vi "GPS.vi"(0 "String":string) -> (1 "Hora":string, 2 "Ubicación":string, 3 "Velocidad":string, 4 "Fecha":string)   [LabVIEW 2020]
doc: "Este programa desglosa las tramas rmc"
panel:
  out "A or V":string
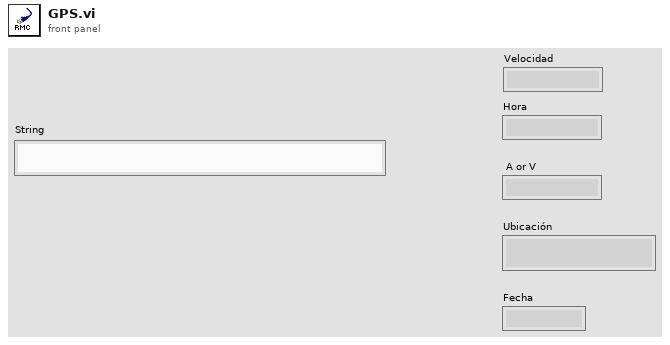
[diagram p1: front panel]
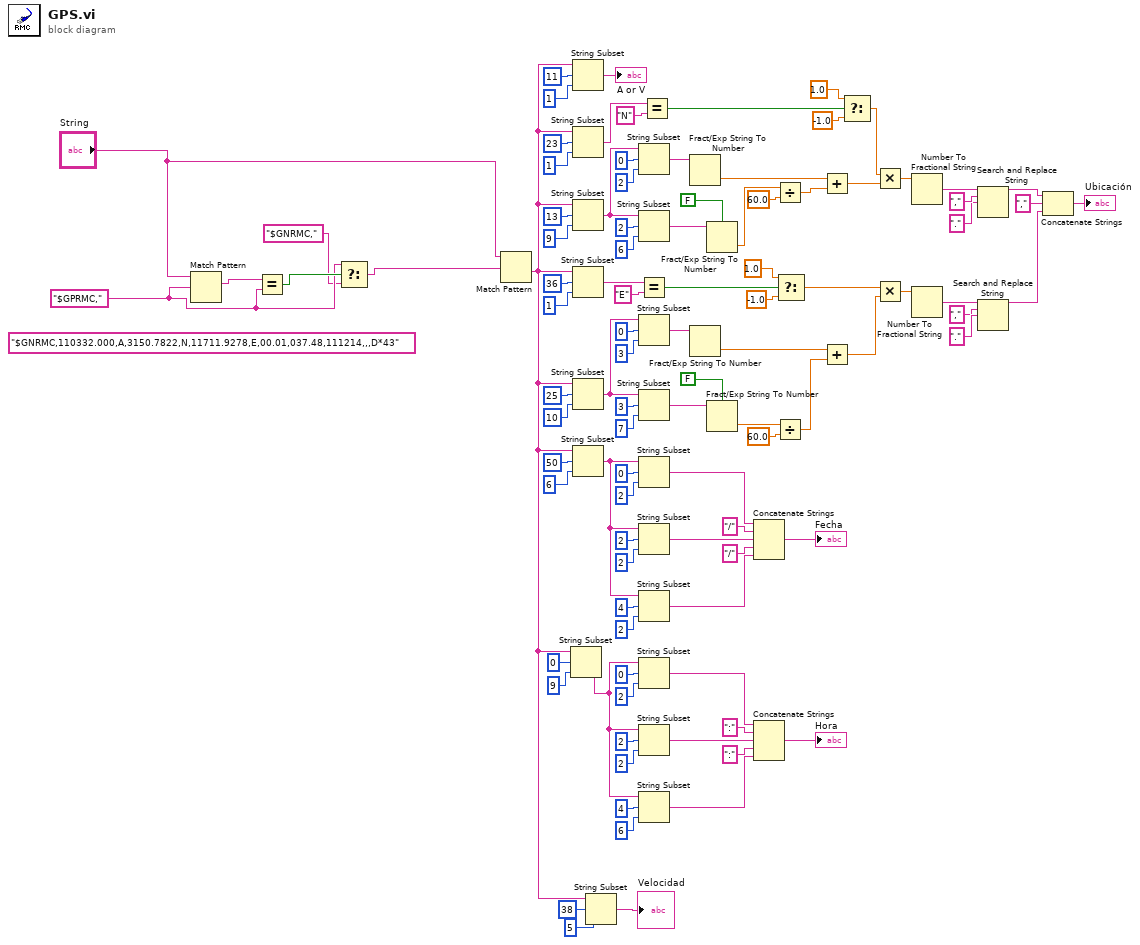
[diagram p0: block diagram]
diagram:
  w4 = "$GPRMC," ("regular expression")
  (unwired) "$GNRMC,110332.000,A,3150.7822,N,11711.9278,E,00.01,037.48,111214,,,D*43"
  n1 = Match Pattern(string="String", regular expression=w4) -> (match substring=w6:string)  [unwired: 1 in, 3 out]
  n2 = Equal?(x=w6, y=w4) -> (x = y?=w5:bool)
  n3 = Select(t=w4, s=w5, f="$GNRMC," ("regular expression")) -> (s? t:f=w2:string)
  n4 = Match Pattern(string="String", regular expression=w2) -> (after substring=w7:string)  [unwired: 1 in, 3 out]
  n5 = String Subset(string=w7, offset (0)=0, length (rest)=9 ("length (rest)")) -> (substring=w35:string)
  n6 = String Subset(string=w7, offset (0)=11, length (rest)=1 ("length (rest)")) -> (substring=→"A or V":string)
  n7 = String Subset(string=w7, offset (0)=23, length (rest)=1 ("length (rest)")) -> (substring=w80:string)
  n8 = String Subset(string=w7, offset (0)=13, length (rest)=9 ("length (rest)")) -> (substring=w92:string)
  n9 = String Subset(string=w7, offset (0)=36, length (rest)=1 ("length (rest)")) -> (substring=w54:string)
  n10 = String Subset(string=w7, offset (0)=25, length (rest)=10 ("length (rest)")) -> (substring=w64:string)
  n11 = String Subset(string=w7, offset (0)=50, length (rest)=6 ("length (rest)")) -> (substring=w19:string)
  n12 = String Subset(string=w7, offset (0)=38, length (rest)=5 ("length (rest)")) -> (substring=→"Velocidad":string)
  n13 = String Subset(string=w92, offset (0)=0, length (rest)=2 ("length (rest)")) -> (substring=w88:string)
  n14 = String Subset(string=w92, offset (0)=2, length (rest)=6 ("length (rest)")) -> (substring=w89:string)
  n15 = Equal?(x=w54, y="E") -> (x = y?=w56:bool)
  n16 = String Subset(string=w64, offset (0)=0, length (rest)=3 ("length (rest)")) -> (substring=w68:string)
  n17 = String Subset(string=w64, offset (0)=3, length (rest)=7 ("length (rest)")) -> (substring=w67:string)
  n18 = String Subset(string=w19, offset (0)=0, length (rest)=2 ("length (rest)")) -> (substring=w16:string)
  n19 = String Subset(string=w19, offset (0)=2, length (rest)=2 ("length (rest)")) -> (substring=w14:string)
  n20 = String Subset(string=w19, offset (0)=4, length (rest)=2 ("length (rest)")) -> (substring=w12:string)
  n21 = String Subset(string=w35, offset (0)=0, length (rest)=2 ("length (rest)")) -> (substring=w32:string)
  n22 = String Subset(string=w35, offset (0)=2, length (rest)=2 ("length (rest)")) -> (substring=w30:string)
  n23 = String Subset(string=w35, offset (0)=4, length (rest)=6 ("length (rest)")) -> (substring=w28:string)
  n24 = Equal?(x=w80, y="N") -> (x = y?=w78:bool)
  n25 = Fract/Exp String To Number(string=w88) -> (number=w84:dbl)  [unwired: 3 in, 1 out]
  n26 = Fract/Exp String To Number(string=w68) -> (number=w72:dbl)  [unwired: 3 in, 1 out]
  n27 = Fract/Exp String To Number(use system decimal point (T)=FALSE, string=w89) -> (number=w86:dbl)  [unwired: 2 in, 1 out]
  n28 = Fract/Exp String To Number(use system decimal point (T)=FALSE, string=w67) -> (number=w70:dbl)  [unwired: 2 in, 1 out]
  n29 = Concatenate Strings(w16, "/" ("string"), w14, "/" ("string"), w12) -> (→"Fecha":string)
  n30 = Concatenate Strings(w32, ":" ("string"), w30, ":" ("string"), w28) -> (→"Hora":string)
  n31 = Divide(x=w86, y=60.0) -> (x/y=w83:dbl)
  n32 = Divide(x=w70, y=60.0) -> (x/y=w73:dbl)
  n33 = Select(t=1.0, s=w56, f=-1.0) -> (s? t:f=w59:dbl)
  n34 = Add(x=w84, y=w83) -> (x+y=w74:dbl)
  n35 = Add(x=w72, y=w73) -> (x+y=w53:dbl)
  n36 = Select(t=1.0, s=w78, f=-1.0) -> (s? t:f=w75:dbl)
  n37 = Multiply(x=w75, y=w74) -> (x*y=w50:dbl)
  n38 = Multiply(x=w59, y=w53) -> (x*y=w49:dbl)
  n39 = Number To Fractional String(number=w50) -> (F-format string=w48:string)  [unwired: 3 in]
  n40 = Number To Fractional String(number=w49) -> (F-format string=w43:string)  [unwired: 3 in]
  n41 = Search and Replace String(input string=w48, search string=",", replace string="." ("replace string (\"\")")) -> (result string=w40:string)  [unwired: 5 in, 3 out]
  n42 = Search and Replace String(input string=w43, search string=",", replace string="." ("replace string (\"\")")) -> (result string=w42:string)  [unwired: 5 in, 3 out]
  n43 = Concatenate Strings(w40, "," ("string"), w42) -> (→"Ubicación":string)
